vi "NavbalLabVIEW(15-5-21).vi"() -> ()   [LabVIEW 2010] (continued)
              n357 = Array Size(array=w4216) -> (size(s)=w4217:i32[])
              n358 = Array Size(array=w4219) -> (size(s)=w4222:i32[])
              n359 = Index Array(array=w4217, index=1) -> (element=w4215:i32)
              n360 = Index Array(array=w4222, index=1) -> (element=w4220:i32)
              n361 = Insert Into Array(array=w4219, index (dim 1)=w4220, new element=w4223) -> (w4210:dbl[][][])  [unwired: 2 in]
              n362 = Insert Into Array(array=w4216, index (dim 1)=w4215, new element=w4214) -> (w4209:dbl[][][])  [unwired: 2 in]
              n363 = Array Size(array=w4210) -> (size(s)=w4213:i32[])
              n364 = Index Array(array=w4213, index=1) -> (element=w4211:i32)
              n365 = Insert Into Array(array=w4210, index (dim 1)=w4211, new element=w4209) -> (w4208:dbl[][][])  [unwired: 2 in]
            }
          }
          n366 = Array Size(array=w3330) -> (size(s)=w3436:i32[])
          n367 = Array Size(array=w3333) -> (size(s)=w3427:i32[])
          n368 = Array Size(array=w3332) -> (size(s)=w3425:i32[])
          n369 = Array Size(array=w3331) -> (size(s)=w3420:i32[])
          n370 = Index Array(array=w3436, index=0) -> (element=w3418:i32)
          n371 = Index Array(array=w3427, index=0) -> (element=w3426:i32)
          n372 = Index Array(array=w3425, index=0) -> (element=w3423:i32)
          n373 = Index Array(array=w3420, index=0) -> (element=w3419:i32)
          n374 = Greater?(x=w3418, y=700) -> (0:w3429:bool)
          n375 = Or(x="Mark Current", y=w3366) -> (x .or. y?=w3367:bool)
          n376 = case shown="True" "Averaging" {
            tunnel: [10 "Number of Averages"] -> w3416
            frame False {
            }
            frame True {
            }
          }
          n377 = case shown="\"Simulated Signals Ohio\"" w3369 {
            tunnel: [w4378 w4427 w4476] -> w3480
            tunnel: [w4382 w4431 w4480] -> w3478
            tunnel: [w4380 w4429 w4478] -> w3523
            tunnel: [w4369 w4424 w4473] -> w3328
            tunnel: [w4381 w4430 w4479] -> w3407
            tunnel: [w4379 w4428 w4477] -> w3406
            tunnel: [w4377 w4426 w4475] -> w3456
            tunnel: [w4376 w4425 w4474] -> w3532
            tunnel: w3530 -> [w4383 w4432 w4481]
            tunnel: w3416 -> [w4370 w4418 w4467]
            frame "Simulated Signals Ohio" {
              # "Ensure that buffer is full before processing"
              # ">>  data out from buffer  >>"
              n378 = local read "Number of Samples"() -> (w4384:i32)
              n379 = call "Convert to Dynamic Data11"("Array"=bool[] [FALSE, FALSE, FALSE, FALSE, FALSE, FALSE, FALSE, FALSE, FALSE, FALSE, TRUE, FALSE, FALSE, FALSE, FALSE, FALSE, FALSE, FALSE, FALSE, FALSE]) -> ("Dynamic Data Type"=w4372:dynamicdata)  [unwired: 3 in]
              n380 = call-poly <userlib>:"Circular Buffer.vi"("Buffer Size"=w4383, "Read Size"=w4384, "Operation"=Circular_Buffer_Operations."Read (most recent)") -> ("Data Out"=w4371:waveform(dbl)[])  [unwired: 5 in, 3 out]
              n381 = call "Select Tach Port2"("Selector Input"=w4372, "Signals"=w4371) -> ("Signal Out"=w4376:dynamicdata)  [unwired: 8 in, 1 out]
              n382 = call "Convert from Dynamic Data49"("Dynamic Data Type"=w4371) -> ("Array"=w4387:dbl[][])  [unwired: 3 in]
              n383 = call "Convert to Dynamic Data10"("Array"=bool[] [TRUE, FALSE, FALSE, FALSE, FALSE, FALSE, FALSE, FALSE, FALSE, FALSE, FALSE, FALSE, FALSE, FALSE, FALSE, FALSE, FALSE, FALSE, FALSE, FALSE]) -> ("Dynamic Data Type"=w4374:dynamicdata)  [unwired: 3 in]
              n384 = Array Size(array=w4387) -> (size(s)=w4390:i32[])
              n385 = call "Select Tach Stbd3"("Selector Input"=w4374, "Signals"=w4371) -> ("Signal Out"=w4369:dynamicdata)  [unwired: 8 in, 1 out]
              n386 = Equal?(x=w4390, y=w4384) -> (x = y?=w4388:bool[])
              n387 = Index Array(array=w4388, index=1) -> (element=w4385:bool)
              n388 = case shown="True" w4385 {
                tunnel: w4371 -> [_ w4410]
                tunnel: [w4391 w4403] -> w4382
                tunnel: [w4393 w4400] -> w4381
                tunnel: [w4391 w4402] -> w4380
                tunnel: [w4391 w4401] -> w4378
                tunnel: [w4393 w4397] -> w4379
                tunnel: [w4393 w4398] -> w4377
                tunnel: w4370 -> [_ w4396]
                frame False {
                  w4391 = cluster{"x0":dbl, "dx":dbl, "magnitude":dbl[]}[] [] ("spectra")
                  n389 = local read "DAQ Start"() -> (w4392:bool)
                  n390 = case shown="True" w4392 {
                    frame False {
                      n391 = property on="DAQ Start" class="Bool (strict)"("BoolText.Text"="DAQ START" ("Boolean Text.Text")) -> ()  [unwired: 2 in, 2 out]
                    }
                    frame True {
                      n392 = property on="DAQ Start" class="Bool (strict)"("BoolText.Text"="Buffering..." ("Boolean Text.Text")) -> ()  [unwired: 2 in, 2 out]
                    }
                  }
                  n393 = local read "Default Stbd Graph"() -> (w4393:dynamicdata)
                }
                frame True {
                  # "convert to VdB"
                  # "convert to VdB"
                  # "convert to VdB"
                  n394 = local read "DAQ Start"() -> (w4399:bool)
                  n395 = case shown="True" w4399 {
                    frame False {
                    }
                    frame True {
                      n396 = property on="DAQ Start" class="Bool (strict)"("BoolText.Text"="DAQ STOP" ("Boolean Text.Text")) -> ()  [unwired: 2 in, 2 out]
                    }
                  }
                  n397 = call "Convert to Dynamic Data3"("Array"=bool[] [FALSE, FALSE, FALSE, FALSE, FALSE, FALSE, FALSE, FALSE, FALSE, FALSE, TRUE, TRUE, TRUE, TRUE, TRUE, TRUE, TRUE, TRUE, TRUE, TRUE]) -> ("Dynamic Data Type"=w4411:dynamicdata)  [unwired: 3 in]
                  n398 = call "Select Port"("Selector Input"=w4411, "Signals"=w4410) -> ("Signal Out"=w4397:dynamicdata)  [unwired: 8 in, 1 out]
                  n399 = call "Convert to Dynamic Data2"("Array"=bool[] [TRUE, TRUE, TRUE, TRUE, TRUE, TRUE, TRUE, TRUE, TRUE, TRUE, FALSE, FALSE, FALSE, FALSE, FALSE, FALSE, FALSE, FALSE, FALSE, FALSE]) -> ("Dynamic Data Type"=w4415:dynamicdata)  [unwired: 3 in]
                  n400 = call "Select Stbd"("Selector Input"=w4415, "Signals"=w4410) -> ("Signal Out"=w4400:dynamicdata)  [unwired: 8 in, 1 out]
                  n401 = call "Convert to Dynamic Data4"("Array"=bool[] [FALSE, FALSE, FALSE, FALSE, FALSE, FALSE, FALSE, FALSE, FALSE, FALSE, FALSE, FALSE, FALSE, FALSE, FALSE, FALSE, FALSE, FALSE, FALSE, FALSE, TRUE, TRUE, TRUE, TRUE, TRUE, TRUE, TRUE, TRUE, TRUE, TRUE, TRUE, TRUE]) -> ("Dynamic Data Type"=w4412:dynamicdata)  [unwired: 3 in]
                  n402 = call "Select Corner"("Selector Input"=w4412, "Signals"=w4410) -> ("Signal Out"=w4398:dynamicdata)  [unwired: 8 in, 1 out]
                  n403 = call-poly <vilib>:"SVL Set dB Reference.vi"("dB reference [EU]"=3.937e-07, "scaled signals in [EU]"=w4400) -> ("scaled signals out [EU]"=w4408:waveform(dbl)[])  [unwired: 8 in, 1 out]
                  n404 = call-poly <vilib>:"SVL Set dB Reference.vi"("dB reference [EU]"=3.937e-07, "scaled signals in [EU]"=w4398) -> ("scaled signals out [EU]"=w4404:waveform(dbl)[])  [unwired: 8 in, 1 out]
                  n405 = call-poly <vilib>:"SVL Set dB Reference.vi"("dB reference [EU]"=3.937e-07, "scaled signals in [EU]"=w4397) -> ("scaled signals out [EU]"=w4406:waveform(dbl)[])  [unwired: 8 in, 1 out]
                  n406 = call "Power Spectrum3"("input signals"=w4406, "number of averages"=w4396) -> ("spectra"=w4402:cluster{"x0":dbl, "dx":dbl, "magnitude":dbl[]}[])  [unwired: 12 in, 5 out]
                  n407 = call "Power Spectrum6"("input signals"=w4404, "number of averages"=w4396) -> ("spectra"=w4401:cluster{"x0":dbl, "dx":dbl, "magnitude":dbl[]}[])  [unwired: 12 in, 5 out]
                  n408 = call "Power Spectrum2"("input signals"=w4408, "number of averages"=w4396) -> ("spectra"=w4403:cluster{"x0":dbl, "dx":dbl, "magnitude":dbl[]}[])  [unwired: 12 in, 5 out]
                }
              }
            }
            frame "LA Class" {
              # "Ensure that buffer is full before processing"
              # ">>  data out from buffer  >>"
              n409 = local read "Number of Samples"() -> (w4433:i32)
              n410 = call "Convert to Dynamic Data19"("Array"=bool[] [FALSE, FALSE, FALSE, FALSE, FALSE, FALSE, FALSE, FALSE, FALSE, FALSE, FALSE, FALSE, FALSE, FALSE, FALSE, FALSE, FALSE, FALSE, FALSE, FALSE, FALSE, FALSE, FALSE, FALSE, FALSE, TRUE]) -> ("Dynamic Data Type"=w4420:dynamicdata)  [unwired: 3 in]
              n411 = call-poly <userlib>:"Circular Buffer.vi"("Buffer Size"=w4432, "Read Size"=w4433, "Operation"=Circular_Buffer_Operations."Read (most recent)") -> ("Data Out"=w4419:waveform(dbl)[])  [unwired: 5 in, 3 out]
              n412 = call "Select Tach Port4"("Selector Input"=w4420, "Signals"=w4419) -> ("Signal Out"=w4425:dynamicdata)  [unwired: 8 in, 1 out]
              n413 = call "Convert from Dynamic Data5"("Dynamic Data Type"=w4419) -> ("Array"=w4436:dbl[][])  [unwired: 3 in]
              n414 = call "Convert to Dynamic Data18"("Array"=bool[] [TRUE, FALSE, FALSE, FALSE, FALSE, FALSE, FALSE, FALSE, FALSE, FALSE, FALSE, FALSE, FALSE, FALSE, FALSE, FALSE, FALSE, FALSE, FALSE, FALSE]) -> ("Dynamic Data Type"=w4422:dynamicdata)  [unwired: 3 in]
              n415 = Array Size(array=w4436) -> (size(s)=w4439:i32[])
              n416 = call "Select Tach Stbd2"("Selector Input"=w4422, "Signals"=w4419) -> ("Signal Out"=w4424:dynamicdata)  [unwired: 8 in, 1 out]
              n417 = Equal?(x=w4439, y=w4433) -> (x = y?=w4437:bool[])
              n418 = Index Array(array=w4437, index=1) -> (element=w4434:bool)
              n419 = case shown="False" w4434 {
                tunnel: w4419 -> [_ w4462]
                tunnel: [w4440 w4455] -> w4431
                tunnel: [w4442 w4452] -> w4430
                tunnel: [w4440 w4454] -> w4429
                tunnel: [w4440 w4453] -> w4427
                tunnel: [w4442 w4449] -> w4428
                tunnel: [w4442 w4450] -> w4426
                tunnel: w4418 -> [_ w4448]
                frame False {
                  w4440 = cluster{"x0":dbl, "dx":dbl, "magnitude":dbl[]}[] [] ("spectra")
                  n420 = local read "DAQ Start"() -> (w4441:bool)
                  n421 = case shown="True" w4441 {
                    frame False {
                      n422 = property on="DAQ Start" class="Bool (strict)"("BoolText.Text"="DAQ START" ("Boolean Text.Text")) -> ()  [unwired: 2 in, 2 out]
                    }
                    frame True {
                      n423 = property on="DAQ Start" class="Bool (strict)"("BoolText.Text"="Buffering..." ("Boolean Text.Text")) -> ()  [unwired: 2 in, 2 out]
                    }
                  }
                  n424 = local read "Default Stbd Graph"() -> (w4442:dynamicdata)
                }
                frame True {
                  # "convert to VdB"
                  # "convert to VdB"
                  # "convert to VdB"
                  n425 = local read "DAQ Start"() -> (w4451:bool)
                  n426 = case shown="True" w4451 {
                    frame False {
                    }
                    frame True {
                      n427 = property on="DAQ Start" class="Bool (strict)"("BoolText.Text"="DAQ STOP" ("Boolean Text.Text")) -> ()  [unwired: 2 in, 2 out]
                    }
                  }
                  n428 = call "Convert to Dynamic Data16"("Array"=bool[] [FALSE, FALSE, FALSE, FALSE, FALSE, FALSE, FALSE, FALSE, FALSE, FALSE, FALSE, FALSE, FALSE, FALSE, FALSE, FALSE, FALSE, FALSE, FALSE, FALSE, FALSE, FALSE, FALSE, FALSE, FALSE, TRUE, TRUE, TRUE, TRUE, TRUE, TRUE, TRUE, TRUE, TRUE, TRUE, TRUE, TRUE, TRUE]) -> ("Dynamic Data Type"=w4463:dynamicdata)  [unwired: 3 in]
                  n429 = call "Select Port3"("Selector Input"=w4463, "Signals"=w4462) -> ("Signal Out"=w4449:dynamicdata)  [unwired: 8 in, 1 out]
                  n430 = call "Convert to Dynamic Data15"("Array"=bool[] [TRUE, FALSE, FALSE, FALSE, FALSE, FALSE, FALSE, FALSE, FALSE, FALSE, FALSE, FALSE, FALSE, TRUE, TRUE, TRUE, TRUE, TRUE, TRUE, TRUE, TRUE, TRUE, TRUE, TRUE, TRUE, FALSE, FALSE, FALSE, FALSE, FALSE, FALSE, FALSE, FALSE, FALSE, FALSE, FALSE, FALSE, FALSE]) -> ("Dynamic Data Type"=w4465:dynamicdata)  [unwired: 3 in]
                  n431 = call "Select Stbd4"("Selector Input"=w4465, "Signals"=w4462) -> ("Signal Out"=w4452:dynamicdata)  [unwired: 8 in, 1 out]
                  n432 = call "Convert to Dynamic Data17"("Array"=bool[] [FALSE, TRUE, TRUE, TRUE, TRUE, TRUE, TRUE, TRUE, TRUE, TRUE, TRUE, TRUE, TRUE, FALSE, FALSE, FALSE, FALSE, FALSE, FALSE, FALSE, FALSE, FALSE, FALSE, FALSE, FALSE, FALSE, FALSE, FALSE, FALSE, FALSE, FALSE, FALSE, FALSE, FALSE, FALSE, FALSE, FALSE, FALSE]) -> ("Dynamic Data Type"=w4464:dynamicdata)  [unwired: 3 in]
                  n433 = call "Select Corner4"("Selector Input"=w4464, "Signals"=w4462) -> ("Signal Out"=w4450:dynamicdata)  [unwired: 8 in, 1 out]
                  n434 = call-poly <vilib>:"SVL Set dB Reference.vi"("dB reference [EU]"=3.937e-07, "scaled signals in [EU]"=w4452) -> ("scaled signals out [EU]"=w4460:waveform(dbl)[])  [unwired: 8 in, 1 out]
                  n435 = call-poly <vilib>:"SVL Set dB Reference.vi"("dB reference [EU]"=3.937e-07, "scaled signals in [EU]"=w4450) -> ("scaled signals out [EU]"=w4456:waveform(dbl)[])  [unwired: 8 in, 1 out]
                  n436 = call-poly <vilib>:"SVL Set dB Reference.vi"("dB reference [EU]"=3.937e-07, "scaled signals in [EU]"=w4449) -> ("scaled signals out [EU]"=w4458:waveform(dbl)[])  [unwired: 8 in, 1 out]
                  n437 = call "Power Spectrum12"("input signals"=w4456, "number of averages"=w4448) -> ("spectra"=w4453:cluster{"x0":dbl, "dx":dbl, "magnitude":dbl[]}[])  [unwired: 12 in, 5 out]
                  n438 = call "Power Spectrum11"("input signals"=w4458, "number of averages"=w4448) -> ("spectra"=w4454:cluster{"x0":dbl, "dx":dbl, "magnitude":dbl[]}[])  [unwired: 12 in, 5 out]
                  n439 = call "Power Spectrum10"("input signals"=w4460, "number of averages"=w4448) -> ("spectra"=w4455:cluster{"x0":dbl, "dx":dbl, "magnitude":dbl[]}[])  [unwired: 12 in, 5 out]
                }
              }
            }
            frame "Ohio Class" {
              # "Ensure that buffer is full before processing"
              # ">>  data out from buffer  >>"
              n440 = local read "Number of Samples"() -> (w4482:i32)
              n441 = call "Convert to Dynamic Data24"("Array"=bool[] [FALSE, FALSE, FALSE, FALSE, FALSE, FALSE, FALSE, FALSE, FALSE, FALSE, FALSE, FALSE, FALSE, FALSE, FALSE, FALSE, FALSE, FALSE, FALSE, FALSE, FALSE, FALSE, TRUE]) -> ("Dynamic Data Type"=w4469:dynamicdata)  [unwired: 3 in]
              n442 = call-poly <userlib>:"Circular Buffer.vi"("Buffer Size"=w4481, "Read Size"=w4482, "Operation"=Circular_Buffer_Operations."Read (most recent)") -> ("Data Out"=w4468:waveform(dbl)[])  [unwired: 5 in, 3 out]
              n443 = call "Select Tach Port5"("Selector Input"=w4469, "Signals"=w4468) -> ("Signal Out"=w4474:dynamicdata)  [unwired: 8 in, 1 out]
              n444 = call "Convert from Dynamic Data6"("Dynamic Data Type"=w4468) -> ("Array"=w4485:dbl[][])  [unwired: 3 in]
              n445 = call "Convert to Dynamic Data23"("Array"=bool[] [TRUE, FALSE, FALSE, FALSE, FALSE, FALSE, FALSE, FALSE, FALSE, FALSE, FALSE, FALSE, FALSE, FALSE, FALSE, FALSE, FALSE, FALSE, FALSE, FALSE]) -> ("Dynamic Data Type"=w4471:dynamicdata)  [unwired: 3 in]
              n446 = Array Size(array=w4485) -> (size(s)=w4488:i32[])
              n447 = call "Select Tach Stbd5"("Selector Input"=w4471, "Signals"=w4468) -> ("Signal Out"=w4473:dynamicdata)  [unwired: 8 in, 1 out]
              n448 = Equal?(x=w4488, y=w4482) -> (x = y?=w4486:bool[])
              n449 = Index Array(array=w4486, index=1) -> (element=w4483:bool)
              n450 = case shown="False" w4483 {
                tunnel: w4468 -> [_ w4508]
                tunnel: [w4489 w4501] -> w4480
                tunnel: [w4491 w4498] -> w4479
                tunnel: [w4489 w4500] -> w4478
                tunnel: [w4489 w4499] -> w4476
                tunnel: [w4491 w4495] -> w4477
                tunnel: [w4491 w4496] -> w4475
                tunnel: w4467 -> [_ w4494]
                frame False {
                  w4489 = cluster{"x0":dbl, "dx":dbl, "magnitude":dbl[]}[] [] ("spectra")
                  n451 = local read "DAQ Start"() -> (w4490:bool)
                  n452 = case shown="True" w4490 {
                    frame False {
                      n453 = property on="DAQ Start" class="Bool (strict)"("BoolText.Text"="DAQ START" ("Boolean Text.Text")) -> ()  [unwired: 2 in, 2 out]
                    }
                    frame True {
                      n454 = property on="DAQ Start" class="Bool (strict)"("BoolText.Text"="Buffering..." ("Boolean Text.Text")) -> ()  [unwired: 2 in, 2 out]
                    }
                  }
                  n455 = local read "Default Stbd Graph"() -> (w4491:dynamicdata)
                }
                frame True {
                  # "convert to VdB"
                  # "convert to VdB"
                  # "convert to VdB"
                  n456 = local read "DAQ Start"() -> (w4497:bool)
                  n457 = case shown="True" w4497 {
                    frame False {
                    }
                    frame True {
                      n458 = property on="DAQ Start" class="Bool (strict)"("BoolText.Text"="DAQ STOP" ("Boolean Text.Text")) -> ()  [unwired: 2 in, 2 out]
                    }
                  }
                  n459 = call "Convert to Dynamic Data21"("Array"=bool[] [FALSE, FALSE, FALSE, FALSE, FALSE, FALSE, FALSE, FALSE, FALSE, FALSE, FALSE, FALSE, FALSE, FALSE, FALSE, FALSE, FALSE, FALSE, FALSE, FALSE, FALSE, FALSE, TRUE, TRUE, TRUE, TRUE, TRUE, TRUE, TRUE, TRUE, TRUE, TRUE]) -> ("Dynamic Data Type"=w4509:dynamicdata)  [unwired: 3 in]
                  n460 = call "Select Port5"("Selector Input"=w4509, "Signals"=w4508) -> ("Signal Out"=w4495:dynamicdata)  [unwired: 8 in, 1 out]
                  n461 = call "Convert to Dynamic Data20"("Array"=bool[] [TRUE, FALSE, FALSE, FALSE, FALSE, FALSE, FALSE, FALSE, FALSE, FALSE, FALSE, FALSE, FALSE, TRUE, TRUE, TRUE, TRUE, TRUE, TRUE, TRUE, TRUE, TRUE]) -> ("Dynamic Data Type"=w4513:dynamicdata)  [unwired: 3 in]
                  n462 = call "Select Stbd5"("Selector Input"=w4513, "Signals"=w4508) -> ("Signal Out"=w4498:dynamicdata)  [unwired: 8 in, 1 out]
                  n463 = call "Convert to Dynamic Data22"("Array"=bool[] [FALSE, TRUE, TRUE, TRUE, TRUE, TRUE, TRUE, TRUE, TRUE, TRUE, TRUE, TRUE, TRUE, FALSE, FALSE, FALSE, FALSE, FALSE, FALSE, FALSE, FALSE, FALSE, FALSE, FALSE, FALSE, FALSE, FALSE, FALSE, FALSE, FALSE, FALSE, FALSE]) -> ("Dynamic Data Type"=w4510:dynamicdata)  [unwired: 3 in]
                  n464 = call "Select Corner5"("Selector Input"=w4510, "Signals"=w4508) -> ("Signal Out"=w4496:dynamicdata)  [unwired: 8 in, 1 out]
                  n465 = call-poly <vilib>:"SVL Set dB Reference.vi"("dB reference [EU]"=3.937e-07, "scaled signals in [EU]"=w4498) -> ("scaled signals out [EU]"=w4506:waveform(dbl)[])  [unwired: 8 in, 1 out]
                  n466 = call-poly <vilib>:"SVL Set dB Reference.vi"("dB reference [EU]"=3.937e-07, "scaled signals in [EU]"=w4496) -> ("scaled signals out [EU]"=w4502:waveform(dbl)[])  [unwired: 8 in, 1 out]
                  n467 = call-poly <vilib>:"SVL Set dB Reference.vi"("dB reference [EU]"=3.937e-07, "scaled signals in [EU]"=w4495) -> ("scaled signals out [EU]"=w4504:waveform(dbl)[])  [unwired: 8 in, 1 out]
                  n468 = call "Power Spectrum15"("input signals"=w4502, "number of averages"=w4494) -> ("spectra"=w4499:cluster{"x0":dbl, "dx":dbl, "magnitude":dbl[]}[])  [unwired: 12 in, 5 out]
                  n469 = call "Power Spectrum13"("input signals"=w4506, "number of averages"=w4494) -> ("spectra"=w4501:cluster{"x0":dbl, "dx":dbl, "magnitude":dbl[]}[])  [unwired: 12 in, 5 out]
                  n470 = call "Power Spectrum14"("input signals"=w4504, "number of averages"=w4494) -> ("spectra"=w4500:cluster{"x0":dbl, "dx":dbl, "magnitude":dbl[]}[])  [unwired: 12 in, 5 out]
                }
              }
            }
          }
          "Default Stbd Graph" <- w3407
          "spectra" <- w3523
          n471 = call "Convert from Dynamic Data48"("Dynamic Data Type"=w3532) -> ("Array"=w3544:dbl[])  [unwired: 3 in]
          n472 = Array Max & Min(array=w3544) -> (max value=w3533:dbl)  [unwired: 3 out]
          n473 = Greater?(x=w3533, y=1.0) -> (0:w3542:bool)
          n474 = case shown="True" w3542 {
            tunnel: w3532 -> [_ w4359]
            tunnel: [0.0 ("detected frequency") w4356] -> w3538
            frame False {
            }
            frame True {
              n475 = call "Filter2"("Signal"=w4359) -> ("Filtered Signal"=w4360:dynamicdata)  [unwired: 9 in, 1 out]
              n476 = call-poly <vilib>:"Extract Single Tone Information.vi"("time signals in"=w4360) -> ("detected frequencies"=w4358:dbl[])  [unwired: 5 in, 5 out]
              n477 = Index Array(array=w4358, index=0) -> (element=w4356:dbl)
            }
          }
          "Frequency (Hz) 2" <- w3538
          n478 = Multiply(x=w3538, y=60.0) -> (x*y=→"Frequency (RPM) 2":dbl)
          n479 = In Range and Coerce(upper limit=60.6, x=w3538, lower limit=60.4) -> (In Range?=w3535:bool)  [unwired: 1 out]
          n480 = case shown="True" w3535 {
            tunnel: [u32 16752008 u32 5308226] -> w3534
            frame False {
            }
            frame True {
            }
          }
          n481 = property on="Frequency (Hz) 2" class="DigNum (strict)"("NumText.BGColor"=w3534) -> ()  [unwired: 2 in, 2 out]
          n482 = property on="Frequency (RPM) 2" class="DigNum (strict)"("NumText.BGColor"=w3534) -> ()  [unwired: 2 in, 2 out]
          n483 = call "Convert from Dynamic Data47"("Dynamic Data Type"=w3328) -> ("Array"=w3554:dbl[])  [unwired: 3 in]
          n484 = Array Max & Min(array=w3554) -> (max value=w3551:dbl)  [unwired: 3 out]
          n485 = Greater?(x=w3551, y=1.0) -> (0:w3552:bool)
          n486 = case shown="True" w3552 {
            tunnel: w3328 -> [_ w4365]
            tunnel: [0.0 ("detected frequency") w4364] -> w3537
            frame False {
            }
            frame True {
              n487 = call "Filter"("Signal"=w4365) -> ("Filtered Signal"=w4366:dynamicdata)  [unwired: 9 in, 1 out]
              n488 = call-poly <vilib>:"Extract Single Tone Information.vi"("time signals in"=w4366) -> ("detected frequencies"=w4367:dbl[])  [unwired: 5 in, 5 out]
              n489 = Index Array(array=w4367, index=0) -> (element=w4364:dbl)
            }
          }
          "Frequency (Hz) 1" <- w3537
          n490 = Multiply(x=w3537, y=60.0) -> (x*y=→"Frequency (RPM) 1":dbl)
          n491 = In Range and Coerce(upper limit=59.6, x=w3537, lower limit=59.4) -> (In Range?=w3549:bool)  [unwired: 1 out]
          n492 = case shown="True" w3549 {
            tunnel: [u32 16752008 u32 5308226] -> w3545
            frame False {
            }
            frame True {
            }
          }
          n493 = property on="Frequency (Hz) 1" class="DigNum (strict)"("NumText.BGColor"=w3545) -> ()  [unwired: 2 in, 2 out]
          n494 = property on="Frequency (RPM) 1" class="DigNum (strict)"("NumText.BGColor"=w3545) -> ()  [unwired: 2 in, 2 out]
          n495 = case shown="True" w3367 {
            frame False {
            }
            frame True {
              n496 = local read "time string"() -> (→"Marker Time":string)
              n497 = local read "Mils/Sec-Phase(CORNERS-Stbd)"() -> (w4242:sgl[][])
              n498 = local read "Mils/Sec-Phase(CORNERS-Port)"() -> (w4245:sgl[][])
              n499 = local read "Mils/Sec-Phase(STBD)"() -> (w4244:dbl[][])
              n500 = local read "Mils/Sec-Phase(PORT)"() -> (w4243:sgl[][])
              n501 = Array Size(array=w4242) -> (size(s)=w4241:i32[])
              n502 = Index Array(array=w4241, index=0) -> (element=w4239:i32)
              n503 = Insert Into Array(array=w4242, index (row)=w4239, new element #1=w4245, new element #2=w4244, new element #3=w4243) -> (w4238:sgl[][])  [unwired: 1 in]
              n504 = local read "Marker Mag"() -> (w4234:sgl[][])
              n505 = local read "Marker Phase"() -> (w4227:sgl[][])
              n506 = Index Array "Mag"(array=w4238, index (col)=0 ("disabled index (col)")) -> (element=w4235:sgl[])  [unwired: 1 in]
              n507 = Index Array "Phase"(array=w4238, index (col)=1 ("disabled index (col)")) -> (element=w4226:sgl[])  [unwired: 1 in]
              n508 = Array Size(array=w4234) -> (size(s)=w4233:i32[])
              n509 = Array Size(array=w4227) -> (size(s)=w4228:i32[])
              n510 = Index Array(array=w4233, index=1) -> (element=w4231:i32)
              n511 = Insert Into Array(array=w4234, index (col)=w4231, new element=w4235) -> (→"Marker Mag":sgl[][])  [unwired: 1 in]
              n512 = Index Array(array=w4228, index=1) -> (element=w4225:i32)
              n513 = Insert Into Array(array=w4227, index (col)=w4225, new element=w4226) -> (→"Marker Phase":sgl[][])  [unwired: 1 in]
            }
          }
          n514 = case shown="True" w3429 {
            tunnel: [w3940 w3944] -> w3434
            tunnel: w3333 -> [w3940 w3957]
            tunnel: [w3939 w3943] -> w3433
            tunnel: w3332 -> [w3939 w3955]
            tunnel: [w3938 w3942] -> w3432
            tunnel: w3331 -> [w3938 w3950]
            tunnel: [w3937 w3941] -> w3431
            tunnel: w3330 -> [w3937 w3948]
            tunnel: w3426 -> [_ w3956]
            tunnel: w3423 -> [_ w3954]
            tunnel: 600 ("y") -> [_ w3945]
            tunnel: w3419 -> [_ w3951]
            tunnel: w3418 -> [_ w3947]
            frame False {
            }
            frame True {
              n515 = Subtract(x=w3956, y=w3945) -> (x-y=w3953:i32)
              n516 = Subtract(x=w3954, y=w3945) -> (x-y=w3952:i32)
              n517 = Subtract(x=w3951, y=w3945) -> (x-y=w3949:i32)
              n518 = Subtract(x=w3947, y=w3945) -> (x-y=w3946:i32)
              n519 = Delete From Array(array=w3957, length=w3953, index (dim 0)=w3945) -> (array with subset deleted=w3944:dbl[][][])  [unwired: 2 in, 1 out]
              n520 = Delete From Array(array=w3955, length=w3952, index (dim 0)=w3945) -> (array with subset deleted=w3943:dbl[][][])  [unwired: 2 in, 1 out]
              n521 = Delete From Array(array=w3950, length=w3949, index (dim 0)=w3945) -> (array with subset deleted=w3942:dbl[][][])  [unwired: 2 in, 1 out]
              n522 = Delete From Array(array=w3948, length=w3946, index (dim 0)=w3945) -> (array with subset deleted=w3941:dbl[][][])  [unwired: 2 in, 1 out]
            }
          }
          n523 = Array Subset(array=w3334, index (dim 0)=0 ("index"), length (dim 0)=600 ("length"), index (dim 1)="DAQ Listbox", length (dim 1)=1 ("length"), index (dim 2)=0 ("index"), length (dim 2)=2 ("length")) -> (w3610:dbl[][][])
          n524 = Array Subset(array=w3334, index (dim 0)=0 ("index"), length (dim 0)=1 ("length"), index (dim 1)="DAQ Listbox", length (dim 1)=1 ("length"), index (dim 2)=0 ("index"), length (dim 2)=2 ("length")) -> (w3595:dbl[][][])
          n525 = Reshape Array(w3610, 600 ("dimension size"), 2 ("dimension size")) -> (w3572:dbl[][])
          n526 = Reshape Array(w3595, 1 ("dimension size"), 2 ("dimension size")) -> (w3582:dbl[][])
          n527 = Index Array(array=w3582, index (col)=0 ("disabled index (col)")) -> (element=w3584:dbl[])  [unwired: 1 in]
          n528 = Index Array(array=w3582, index (col)=1 ("disabled index (col)")) -> (element=w3581:dbl[])  [unwired: 1 in]
          n529 = Array Subset(array=w3572, index (row)=0 ("index"), length (row)=600 ("length"), index (col)=0 ("index"), length (col)=1 ("length")) -> (w3573:dbl[][])
          n530 = Array Subset(array=w3572, index (row)=0 ("index"), length (row)=600 ("length"), index (col)=1 ("index"), length (col)=1 ("length")) -> (w3597:dbl[][])
          n531 = Reshape Array(w3584, 1 ("dimension size")) -> (w3585:dbl[])
          n532 = Reshape Array(w3581, 1 ("dimension size")) -> (w3591:dbl[])
          n533 = Index Array(array=w3585, index=0) -> (element=w3579:dbl)
          n534 = Index Array(array=w3591, index=0) -> (element=w3616:dbl)
          n535 = Reshape Array(w3597, 600 ("dimension size")) -> (w3576:dbl[])
          n536 = Reshape Array(w3573, 600 ("dimension size")) -> (w3580:dbl[])
          n537 = Insert Into Array(array=w3580, index=0, new element=w3579) -> (→"mag":dbl[])
          n538 = Insert Into Array(array=w3576, index=0, new element=w3616) -> (→"phase":dbl[])
          n539 = property on="Tab 3" class="TabCtl (strict)"() -> ("Visible"=w3443:bool)  [unwired: 2 in, 2 out]
          n540 = property on="Tab 3" class="TabCtl (strict)"() -> ("Value"=w3446:T9)  [unwired: 2 in, 2 out]
          n541 = Equal?(x=w3446, y=T19."Step 6: Polar Plots") -> (x = y?=w3444:bool)
          n542 = And(x=w3444, y=w3443) -> (x .and. y?=w3442:bool)
          n543 = case shown="True" w3442 {
            frame False {
            }
            frame True {
              w3989 = 0 ("index")
              w4002 = T21."Application Font" ("desired font(Application)")
              w4004 = cluster{"width":i16, "height":i16} {"width"=575, "height"=575} ("dimensions (w,h)")
              # "Find the max magnitude to be plotted,\nand adjust the scaling of all plots"
              # "Add Corresponding Prediction measurement to Polar plot"
              # "Add Corresponding Baseline measurement to Polar plot"
              # "Polar Plot"
              n544 = local read "Marker Phase"() -> (w3970:sgl[][])
              n545 = local read "Pred plot"() -> (w3958:dbl[][])
              n546 = local read "Marker Mag"() -> (w3963:sgl[][])
              n547 = Array Size(array=w3963) -> (size(s)=w3966:i32[])
              n548 = local read "Ref Pt Plot"() -> (w3976:sgl[][])
              n549 = Index Array(array=w3966, index=1) -> (element=w3964:i32)
              n550 = local read "DAQ Listbox"() -> (w3969:i32)
              n551 = Index Array(array=w3958, index (col)=1 ("disabled index (col)")) -> (element=w3959:dbl[])  [unwired: 1 in]
              n552 = Index Array(array=w3958, index (col)=0 ("disabled index (col)")) -> (element=w3960:dbl[])  [unwired: 1 in]
              n553 = for {
                N: w3964 -> [_]
                tunnel: [w4013] -> w3968
                tunnel: [w4015] -> w3967 mode=indexing
                tunnel: w3969 -> [w4014]
                tunnel: w3970 -> [w4008]
                tunnel: w3963 -> [w4007]
                i -> [w4011]
                n554 = Index Array(array=w4007, index (row)=w4014) -> (element=w4013:sgl[])  [unwired: 1 in]
                n555 = Index Array(array=w4008, index (row)=w4014) -> (element=w4012:sgl[])  [unwired: 1 in]
                n556 = Index Array(array=w4012, index=w4011) -> (element=w4009:sgl)
                n557 = Index Array(array=w4013, index=w4011) -> (element=w4010:sgl)
                n558 = Bundle(w4010, w4009) -> (w4015:cluster{sgl, sgl})  [unwired: 1 in]
              }
              n559 = Index Array(array=w3976, index (col)=0 ("disabled index (col)")) -> (element=w3978:sgl[])  [unwired: 1 in]
              n560 = Index Array(array=w3976, index (col)=1 ("disabled index (col)")) -> (element=w3975:sgl[])  [unwired: 1 in]
              n561 = Index Array(array=w3959, index=w3969) -> (element=w3991:dbl)
              n562 = Index Array(array=w3960, index=w3969) -> (element=w3988:dbl)
              n563 = for {
                N: 600 -> [_]
                tunnel: [w4020] -> w4003 mode=indexing
                i -> [w4021]
                n564 = local read "phase"() -> (w4016:dbl[])
                n565 = local read "mag"() -> (w4017:dbl[])
                n566 = Index Array(array=w4017, index=w4021) -> (element=w4019:dbl)
                n567 = Index Array(array=w4016, index=w4021) -> (element=w4018:dbl)
                n568 = Bundle("mag. (Vpeak)"=w4019, "mag. (Vpeak)"=w4018) -> (w4020:cluster{"mag. (Vpeak)":dbl, "mag. (Vpeak)":dbl})  [unwired: 1 in]
              }
              n569 = local read "mag"() -> (w3994:dbl[])
              n570 = Bundle("Real Matrix Element"=w3988, "Real Matrix Element"=w3991) -> (w3983:T22)  [unwired: 1 in]
              n571 = Index Array(array=w3978, index=w3969) -> (element=w3993:sgl)
              n572 = Index Array(array=w3975, index=w3969) -> (element=w3997:sgl)
              n573 = Insert Into Array(array=w3994, index=w3989, new element #1=w3993, new element #2=0 ("new element/subarray"), new element #3=w3968) -> (w3990:dbl[])
              n574 = Bundle(w3993, w3997) -> (w3996:cluster{sgl, sgl})  [unwired: 1 in]
              n575 = Initialize Array(w3983, 1 ("dimension size")) -> (w3982:T23)
              n576 = Initialize Array(w3996, 1 ("dimension size")) -> (w3992:cluster{sgl, sgl}[])
              n577 = Insert Into Array(array=w3990, index=w3989, new element=w3988) -> (w3987:dbl[])
              n578 = Array Max & Min(array=w3987) -> (max value=w3980:dbl)  [unwired: 3 out]
              n579 = Divide(x=w3980, y=0.9) -> (x/y=w3971:dbl)
              n580 = property on="maximum" class="DigNum (strict)"("Val(Sgnl)"=w3971) -> ()  [unwired: 2 in, 2 out]
              n581 = call <vilib>:"Polar Plot(points&line).vi"("polar attributes"="polar attributes", "desired font(Application)"=w4002, "dimensions (w,h)"=w4004, "data array [mag, phase (deg)]"=w4003) -> ("new picture"=w3999:picture)  [unwired: 7 in]
              n582 = property on="maximum" class="DigNum (strict)"("Val(Sgnl)"=w3971) -> ()  [unwired: 2 in, 2 out]
              n583 = property on="maximum" class="DigNum (strict)"("Val(Sgnl)"=w3971) -> ()  [unwired: 2 in, 2 out]
              n584 = property on="maximum" class="DigNum (strict)"("Val(Sgnl)"=w3971) -> ()  [unwired: 2 in, 2 out]
              n585 = feedback #1() -> (w3998:picture)  [unwired: 1 in]
              n586 = call <vilib>:"Polar Plot(points&line).vi"("polar attributes"="polar attributes Prediction", "desired font(Application)"=w4002, "dimensions (w,h)"=w4004, "data array [mag, phase (deg)]"=w3982, "picture"=w3998) -> ("new picture"=w3986:picture)  [unwired: 6 in]
              n587 = call <vilib>:"Polar Plot(points&line).vi"("polar attributes"="polar attributes Start Point", "desired font(Application)"=w4002, "dimensions (w,h)"=w4004, "data array [mag, phase (deg)]"=w3992, "picture"=w3986) -> ("new picture"=w3973:picture)  [unwired: 6 in]
              n588 = call <vilib>:"Polar Plot(points&line).vi"("polar attributes"="polar attributes Marker", "desired font(Application)"=w4002, "dimensions (w,h)"=w4004, "data array [mag, phase (deg)]"=w3967, "picture"=w3973) -> ("new picture"=→"Polar Plot Picture":picture)  [unwired: 6 in]
              n589 = feedback-in #1(w3999) -> ()
            }
          }
          n590 = local read "Ship Class"() -> (w3555:T4)
          n591 = local read "Frequency (Hz) 1"() -> (w3556:dbl)
          n592 = case shown="\"LA Class\"" w3555 {
            tunnel: w3407 -> [w4856 w4871 w4872]
            tunnel: [w4842 w4857 w4874] -> w3457
            tunnel: [w4855 w4870 w4873] -> w3477
            frame "LA Class" {
              n593 = Split Signals(w4856) -> (w4855:dynamicdata, w4854:dynamicdata, w4853:dynamicdata, w4852:dynamicdata, w4851:dynamicdata, w4850:dynamicdata, w4849:dynamicdata, w4848:dynamicdata, w4847:dynamicdata, w4846:dynamicdata, w4845:dynamicdata, w4844:dynamicdata, w4843:dynamicdata)  [unwired: 13 in]
              n594 = Merge Signals(w4854, w4853, w4852, w4851, w4850, w4849, w4848, w4847, w4846, w4845, w4844, w4843) -> (w4842:dynamicdata)
            }
            frame "Ohio Class" {
              n595 = Split Signals(w4871) -> (w4870:dynamicdata, w4869:dynamicdata, w4868:dynamicdata, w4867:dynamicdata, w4866:dynamicdata, w4865:dynamicdata, w4864:dynamicdata, w4863:dynamicdata, w4862:dynamicdata, w4861:dynamicdata, w4860:dynamicdata, w4859:dynamicdata, w4858:dynamicdata)  [unwired: 13 in]
              n596 = Merge Signals(w4869, w4868, w4867, w4866, w4865, w4864, w4863, w4862, w4861, w4860, w4859, w4858) -> (w4857:dynamicdata)
            }
            frame "Simulated Signals Ohio" {
              n597 = Split Signals(w4872) -> (w4873:dynamicdata, w4875:dynamicdata, w4876:dynamicdata, w4877:dynamicdata, w4878:dynamicdata, w4879:dynamicdata, w4880:dynamicdata, w4881:dynamicdata, w4882:dynamicdata, w4883:dynamicdata)  [unwired: 10 in]
              n598 = Merge Signals(w4875, w4876, w4877, w4878, w4879, w4880, w4881, w4882, w4883) -> (w4874:dynamicdata)
            }
          }
          n599 = local read "Sample Frequency (Hz)"() -> (w3528:i32)
          n600 = local read "Sample Frequency (Hz)"() -> (w3529:i32)
          n601 = local read "Sample Frequency (Hz)"() -> (w3527:i32)
          n602 = local read "Sample Frequency (Hz)"() -> (w3482:i32)
          n603 = case shown="\"Simulated Signals Ohio\"" w3555 {
            tunnel: w3406 -> [w4803 w4826 w4841]
            tunnel: [w4802 w4812 w4827] -> w3665
            tunnel: [w4801 w4825 w4840] -> w3666
            frame "Simulated Signals Ohio" {
              n604 = Split Signals(w4803) -> (w4801:dynamicdata, w4804:dynamicdata, w4805:dynamicdata, w4806:dynamicdata, w4807:dynamicdata, w4808:dynamicdata, w4809:dynamicdata, w4810:dynamicdata, w4811:dynamicdata, w4800:dynamicdata)  [unwired: 10 in]
              n605 = Merge Signals(w4804, w4805, w4806, w4807, w4808, w4809, w4810, w4811, w4800) -> (w4802:dynamicdata)
            }
            frame "LA Class" {
              n606 = Split Signals(w4826) -> (w4825:dynamicdata, w4824:dynamicdata, w4823:dynamicdata, w4822:dynamicdata, w4821:dynamicdata, w4820:dynamicdata, w4819:dynamicdata, w4818:dynamicdata, w4817:dynamicdata, w4816:dynamicdata, w4815:dynamicdata, w4814:dynamicdata, w4813:dynamicdata)  [unwired: 13 in]
              n607 = Merge Signals(w4824, w4823, w4822, w4821, w4820, w4819, w4818, w4817, w4816, w4815, w4814, w4813) -> (w4812:dynamicdata)
            }
            frame "Ohio Class" {
              n608 = Split Signals(w4841) -> (w4840:dynamicdata, w4839:dynamicdata, w4838:dynamicdata, w4837:dynamicdata, w4836:dynamicdata, w4835:dynamicdata, w4834:dynamicdata, w4833:dynamicdata, w4832:dynamicdata, w4831:dynamicdata, w4830:dynamicdata, w4829:dynamicdata, w4828:dynamicdata)  [unwired: 13 in]
              n609 = Merge Signals(w4839, w4838, w4837, w4836, w4835, w4834, w4833, w4832, w4831, w4830, w4829, w4828) -> (w4827:dynamicdata)
            }
          }
          n610 = local read "Frequency (Hz) 2"() -> (w3557:dbl)
          n611 = local read "Frequency (Hz) 1"() -> (w3643:dbl)
          n612 = local read "Frequency (Hz) 2"() -> (w3483:dbl)
          n613 = Array Size(array=w3523) -> (size(s)=w3520:i32)
          n614 = Array Size(array=w3478) -> (size(s)=w3531:i32)
          n615 = Decrement(x=w3520) -> (x-1=w3519:i32)
          n616 = Decrement(x=w3531) -> (x-1=w3521:i32)
          n617 = Array Size(array=w3480) -> (size(s)=w3571:i32)
          n618 = Array Size(array=w3480) -> (size(s)=w3481:i32)
          n619 = for "Phase (Degrees)" {
            N: w3519 -> [_]
            tunnel: w3406 -> [w4979]
            tunnel: [w4981] -> w3691 mode=indexing
            tunnel: w3528 -> [w4980]
            i -> [w4984]
            n620 = Add(x=1, y=w4984) -> (x+y=w4982:i32)
            n621 = call "Convert from Dynamic Data30"("Dynamic Data Type"=w4979, "Channel"=w4982) -> ("Array"=w4987:dbl[])  [unwired: 2 in]
            n622 = call "Convert from Dynamic Data31"("Dynamic Data Type"=w4979, "Channel"=0) -> ("Array"=w4985:dbl[])  [unwired: 2 in]
            n623 = Reciprocal(x=w4980) -> (1/x=w4991:dbl)
            n624 = call <vilib>:"Cross Power Spectrum.vi"("dt"=w4991, "Signal Y (V)"=w4987, "Signal X (V)"=w4985) -> ("Cross Power XY Spectrum Phase (radians)"=w4978:dbl[])  [unwired: 2 out]
            n625 = Divide(x=180, y=3.141592653589793) -> (x/y=w4988:dbl)
            n626 = Multiply(x=w4978, y=w4988) -> (x*y=w4981:dbl[])
          }
          n627 = for "Magnitude (VdB)" {
            N: w3521 -> [_]
            tunnel: w3478 -> [w5053]
            tunnel: [w5049] -> w3704 mode=indexing
            i -> [w5052]
            n628 = Add(x=1, y=w5052) -> (x+y=w5050:i32)
            n629 = Index Array(array=w5053, index=w5050) -> (element=w5054:cluster{"x0":dbl, "dx":dbl, "magnitude":dbl[]})
            n630 = Unbundle(w5054) -> ("magnitude"=w5049:dbl[])  [unwired: 2 out]
          }
          n631 = Index Array(array=w3478) -> (element=w3705:cluster{"x0":dbl, "dx":dbl, "magnitude":dbl[]})  [unwired: 1 in]
          n632 = for "Phase (Degrees)" {
            N: w3521 -> [_]
            tunnel: w3407 -> [w5091]
            tunnel: [w5087] -> w3559 mode=indexing
            tunnel: w3529 -> [w5085]
            i -> [w5089]
            n633 = Add(x=1, y=w5089) -> (x+y=w5086:i32)
            n634 = call "Convert from Dynamic Data27"("Dynamic Data Type"=w5091, "Channel"=w5086) -> ("Array"=w5093:dbl[])  [unwired: 2 in]
            n635 = call "Convert from Dynamic Data28"("Dynamic Data Type"=w5091, "Channel"=0) -> ("Array"=w5090:dbl[])  [unwired: 2 in]
            n636 = Reciprocal(x=w5085) -> (1/x=w5098:dbl)
            n637 = call <vilib>:"Cross Power Spectrum.vi"("dt"=w5098, "Signal Y (V)"=w5093, "Signal X (V)"=w5090) -> ("Cross Power XY Spectrum Phase (radians)"=w5097:dbl[])  [unwired: 2 out]
            n638 = Divide(x=180, y=3.141592653589793) -> (x/y=w5094:dbl)
            n639 = Multiply(x=w5097, y=w5094) -> (x*y=w5087:dbl[])
          }
          n640 = for "Magnitude (VdB)" {
            N: w3519 -> [_]
            tunnel: w3523 -> [w4945]
            tunnel: [w4941] -> w3689 mode=indexing
            i -> [w4944]
            n641 = Add(x=1, y=w4944) -> (x+y=w4942:i32)
            n642 = Index Array(array=w4945, index=w4942) -> (element=w4946:cluster{"x0":dbl, "dx":dbl, "magnitude":dbl[]})
            n643 = Unbundle(w4946) -> ("magnitude"=w4941:dbl[])  [unwired: 2 out]
          }
          n644 = Index Array(array=w3523) -> (element=w3690:cluster{"x0":dbl, "dx":dbl, "magnitude":dbl[]})  [unwired: 1 in]
          n645 = for "Magnitude (VdB)" {
            N: w3571 -> [_]
            tunnel: w3480 -> [w4754]
            tunnel: [w4753] -> w3662 mode=indexing
            i -> [w4752]
            n646 = Index Array(array=w4754, index=w4752) -> (element=w4755:cluster{"x0":dbl, "dx":dbl, "magnitude":dbl[]})
            n647 = Unbundle(w4755) -> ("magnitude"=w4753:dbl[])  [unwired: 2 out]
          }
          n648 = Unbundle(w3705) -> ("dx"=w3703:dbl)  [unwired: 2 out]
          "frequency resolution" <- w3703
          n649 = Index Array(array=w3480) -> (element=w3663:cluster{"x0":dbl, "dx":dbl, "magnitude":dbl[]})  [unwired: 1 in]
          n650 = for "Phase (Degrees)" {
            N: w3571 -> [_]
            tunnel: w3456 -> [w4792]
            tunnel: [w4790] -> w3664 mode=indexing
            tunnel: w3407 -> [w4788]
            tunnel: w3527 -> [w4787]
            i -> [w4789]
            n651 = call "Convert from Dynamic Data33"("Dynamic Data Type"=w4792, "Channel"=w4789) -> ("Array"=w4794:dbl[])  [unwired: 2 in]
            n652 = call "Convert from Dynamic Data34"("Dynamic Data Type"=w4788, "Channel"=0) -> ("Array"=w4791:dbl[])  [unwired: 2 in]
            n653 = Reciprocal(x=w4787) -> (1/x=w4799:dbl)
            n654 = call <vilib>:"Cross Power Spectrum.vi"("dt"=w4799, "Signal Y (V)"=w4794, "Signal X (V)"=w4791) -> ("Cross Power XY Spectrum Phase (radians)"=w4798:dbl[])  [unwired: 2 out]
            n655 = Divide(x=180, y=3.141592653589793) -> (x/y=w4795:dbl)
            n656 = Multiply(x=w4798, y=w4795) -> (x*y=w4790:dbl[])
          }
          n657 = Unbundle(w3690) -> ("dx"=w3688:dbl)  [unwired: 2 out]
          n658 = for "Magnitude (VdB)" {
            N: w3481 -> [_]
            tunnel: w3480 -> [w4307]
            tunnel: [w4306] -> w3513 mode=indexing
            i -> [w4305]
            n659 = Index Array(array=w4307, index=w4305) -> (element=w4308:cluster{"x0":dbl, "dx":dbl, "magnitude":dbl[]})
            n660 = Unbundle(w4308) -> ("magnitude"=w4306:dbl[])  [unwired: 2 out]
          }
          n661 = Index Array(array=w3480) -> (element=w3514:cluster{"x0":dbl, "dx":dbl, "magnitude":dbl[]})  [unwired: 1 in]
          n662 = for "Phase (Degrees)" {
            N: w3481 -> [_]
            tunnel: w3456 -> [w4345]
            tunnel: [w4343] -> w3515 mode=indexing
            tunnel: w3406 -> [w4341]
            tunnel: w3482 -> [w4340]
            i -> [w4342]
            n663 = call "Convert from Dynamic Data"("Dynamic Data Type"=w4345, "Channel"=w4342) -> ("Array"=w4347:dbl[])  [unwired: 2 in]
            n664 = call "Convert from Dynamic Data2"("Dynamic Data Type"=w4341, "Channel"=0) -> ("Array"=w4344:dbl[])  [unwired: 2 in]
            n665 = Reciprocal(x=w4340) -> (1/x=w4352:dbl)
            n666 = call <vilib>:"Cross Power Spectrum.vi"("dt"=w4352, "Signal Y (V)"=w4347, "Signal X (V)"=w4344) -> ("Cross Power XY Spectrum Phase (radians)"=w4351:dbl[])  [unwired: 2 out]
            n667 = Divide(x=180, y=3.141592653589793) -> (x/y=w4348:dbl)
            n668 = Multiply(x=w4351, y=w4348) -> (x*y=w4343:dbl[])
          }
          n669 = Unbundle(w3663) -> ("dx"=w3661:dbl)  [unwired: 2 out]
          "frequency (resolution) corner" <- w3661
          n670 = Unbundle(w3514) -> ("dx"=w3512:dbl)  [unwired: 2 out]
          "frequency (resolution) corners-port" <- w3512
          n671 = for "Mag (VdB)(8x)" {
            N: w3521 -> [_]
            tunnel: w3704 -> [w5035]
            tunnel: w3703 -> [w5033]
            tunnel: w3556 -> [w5031]
            tunnel: [w5030] -> w3696 mode=indexing
            i -> [w5032]
            n672 = Index Array(array=w5035, index (row)=w5032) -> (element=w5029:dbl[])  [unwired: 1 in]
            n673 = for {
              N: 8 -> [_]
              tunnel: [w5040] -> w5030 mode=indexing
              tunnel: w5029 -> [w5044]
              tunnel: w5031 -> [w5046]
              tunnel: w5033 -> [w5048]
              i -> [w5045]
              w5038 = ext 2.0  # change
              n674 = Divide(x=w5046, y=w5048) -> (x/y=w5036:dbl)
              n675 = Multiply(x=w5036, y=w5045) -> (x*y=w5047:dbl)
              n676 = Add(x=w5036, y=w5047) -> (x+y=w5042:dbl)
              n677 = Subtract(x=w5042, y=w5038) -> (x-y=w5043:ext)
              n678 = Multiply(x=w5038, y=2.0) -> (x*y=w5037:ext)
              n679 = Array Subset(array=w5044, index=w5043, length=w5037) -> (w5041:dbl[])
              n680 = Array Max & Min(array=w5041) -> (max value=w5040:dbl)  [unwired: 3 out]
            }
          }
          "Magnitude VdB Stbd" <- w3696
          n681 = for "Mag (VdB)(8x)" {
            N: w3519 -> [_]
            tunnel: w3689 -> [w4927]
            tunnel: w3688 -> [w4925]
            tunnel: w3557 -> [w4923]
            tunnel: [w4922] -> w3681 mode=indexing
            i -> [w4924]
            n682 = Index Array(array=w4927, index (row)=w4924) -> (element=w4921:dbl[])  [unwired: 1 in]
            n683 = for {
              N: 8 -> [_]
              tunnel: [w4932] -> w4922 mode=indexing
              tunnel: w4921 -> [w4936]
              tunnel: w4923 -> [w4938]
              tunnel: w4925 -> [w4940]
              i -> [w4937]
              w4930 = ext 2.0  # change
              n684 = Divide(x=w4938, y=w4940) -> (x/y=w4928:dbl)
              n685 = Multiply(x=w4928, y=w4937) -> (x*y=w4939:dbl)
              n686 = Add(x=w4928, y=w4939) -> (x+y=w4934:dbl)
              n687 = Subtract(x=w4934, y=w4930) -> (x-y=w4935:ext)
              n688 = Multiply(x=w4930, y=2.0) -> (x*y=w4929:ext)
              n689 = Array Subset(array=w4936, index=w4935, length=w4929) -> (w4933:dbl[])
              n690 = Array Max & Min(array=w4933) -> (max value=w4932:dbl)  [unwired: 3 out]
            }
          }
          "Magnitude VdB Port" <- w3681
          n691 = for "Mag (VdB)(8x)" {
            N: w3571 -> [_]
            tunnel: w3662 -> [w4739]
            tunnel: w3661 -> [w4737]
            tunnel: w3643 -> [w4735]
            tunnel: [w4734] -> w3644 mode=indexing
            i -> [w4736]
            n692 = Index Array(array=w4739, index (row)=w4736) -> (element=w4733:dbl[])  [unwired: 1 in]
            n693 = for {
              N: 8 -> [_]
              tunnel: [w4745] -> w4734 mode=indexing
              tunnel: w4733 -> [w4747]
              tunnel: w4735 -> [w4749]
              tunnel: w4737 -> [w4751]
              i -> [w4748]
              # "Encompass wider span\nto ensure max capture"
              n694 = Divide(x=w4749, y=w4751) -> (x/y=w4743:dbl)
              n695 = Multiply(x=w4743, y=w4748) -> (x*y=w4750:dbl)
              n696 = Add(x=w4743, y=w4750) -> (x+y=w4742:dbl)
              n697 = Subtract(x=w4742, y=1 ("length")) -> (x-y=w4740:dbl)
              n698 = Array Subset(array=w4747, index=w4740, length=3) -> (w4746:dbl[])
              n699 = Array Max & Min(array=w4746) -> (max value=w4745:dbl)  [unwired: 3 out]
            }
          }
          "Magnitude VdB Corner" <- w3644
          n700 = for "Mag (VdB)(8x)" {
            N: w3481 -> [_]
            tunnel: w3513 -> [w4290]
            tunnel: w3512 -> [w4288]
            tunnel: w3483 -> [w4286]
            tunnel: [w4285] -> w3495 mode=indexing
            i -> [w4287]
            n701 = Index Array(array=w4290, index (row)=w4287) -> (element=w4284:dbl[])  [unwired: 1 in]
            n702 = for {
              N: 8 -> [_]
              tunnel: [w4298] -> w4285 mode=indexing
              tunnel: w4284 -> [w4300]
              tunnel: w4286 -> [w4302]
              tunnel: w4288 -> [w4304]
              i -> [w4301]
              n703 = Divide(x=w4302, y=w4304) -> (x/y=w4297:dbl)
              n704 = Multiply(x=w4297, y=w4301) -> (x*y=w4303:dbl)
              n705 = Subtract(x=w4297, y=1.0) -> (x-y=w4295:dbl)
              n706 = Add(x=w4295, y=w4303) -> (x+y=w4292:dbl)
              n707 = Subtract(x=w4292, y=1 ("length")) -> (x-y=w4291:dbl)
              n708 = Array Subset(array=w4300, index=w4291, length=3) -> (w4299:dbl[])
              n709 = Array Max & Min(array=w4299) -> (max value=w4298:dbl)  [unwired: 3 out]
            }
          }
          "Magnitude VdB Corners-Port" <- w3495
          n710 = for "Phase (8x)" {
            N: w3521 -> [_]
            tunnel: w3559 -> [w5061]
            tunnel: [w5057] -> w3558 mode=indexing
            tunnel: w3556 -> [w5056]
            tunnel: w3703 -> [w5055]
            i -> [w5058]
            n711 = Index Array(array=w5061, index (row)=w5058) -> (element=w5059:dbl[])  [unwired: 1 in]
            n712 = for {
              N: 8 -> [_]
              tunnel: [w5067] -> w5057 mode=indexing
              tunnel: w5059 -> [w5069]
              tunnel: w5056 -> [w5065]
              tunnel: w5055 -> [w5064]
              i -> [w5070]
              n713 = Divide(x=w5065, y=w5064) -> (x/y=w5063:dbl)
              n714 = Multiply(x=w5063, y=w5070) -> (x*y=w5071:dbl)
              n715 = Add(x=w5063, y=w5071) -> (x+y=w5068:dbl)
              n716 = Index Array(array=w5069, index=w5068) -> (element=w5062:dbl)
              n717 = case shown="\"navbal\"" "phase data format" {
                tunnel: w5062 -> [w5076 w5079 w5084]
                tunnel: [w5072 w5078 w5084] -> w5067
                frame "0-360" {
                  n718 = Negate(x=w5076) -> (-x=w5074:dbl)
                  n719 = Less Than 0?(x=w5076) -> (x < 0?=w5077:bool)
                  n720 = Add(x=w5074, y=180.0) -> (x+y=w5073:dbl)
                  n721 = Select(t=w5073, s=w5077, f=w5076) -> (s? t:f=w5072:dbl)
                }
                frame "navbal" {
                  n722 = Negate(x=w5079) -> (-x=w5083:dbl)
                  n723 = Less Than 0?(x=w5079) -> (x < 0?=w5082:bool)
                  n724 = Subtract(x=360.0, y=w5079) -> (x-y=w5081:dbl)
                  n725 = Select(t=w5083, s=w5082, f=w5081) -> (s? t:f=w5078:dbl)
                }
                frame "pass through", Default {
                }
              }
            }
          }
          "Phase Stbd" <- w3558
          n726 = local read "phase data format"() -> (w3517:string)
          n727 = for "Phase (8x)" {
            N: w3519 -> [_]
            tunnel: w3691 -> [w4954]
            tunnel: [w4950] -> w3415 mode=indexing
            tunnel: w3557 -> [w4949]
            tunnel: w3688 -> [w4948]
            tunnel: w3517 -> [w4947]
            i -> [w4951]
            n728 = Index Array(array=w4954, index (row)=w4951) -> (element=w4952:dbl[])  [unwired: 1 in]
            n729 = for {
              N: 8 -> [_]
              tunnel: [w4959] -> w4950 mode=indexing
              tunnel: w4952 -> [w4962]
              tunnel: w4949 -> [w4958]
              tunnel: w4948 -> [w4957]
              tunnel: w4947 -> [w4955]
              i -> [w4963]
              n730 = Divide(x=w4958, y=w4957) -> (x/y=w4956:dbl)
              n731 = Multiply(x=w4956, y=w4963) -> (x*y=w4964:dbl)
              n732 = Add(x=w4956, y=w4964) -> (x+y=w4961:dbl)
              n733 = Index Array(array=w4962, index=w4961) -> (element=w4960:dbl)
              n734 = case shown="\"navbal\"" w4955 {
                tunnel: w4960 -> [w4969 w4972 w4977]
                tunnel: [w4965 w4971 w4977] -> w4959
                frame "0-360" {
                  n735 = Negate(x=w4969) -> (-x=w4967:dbl)
                  n736 = Less Than 0?(x=w4969) -> (x < 0?=w4970:bool)
                  n737 = Add(x=w4967, y=180.0) -> (x+y=w4966:dbl)
                  n738 = Select(t=w4966, s=w4970, f=w4969) -> (s? t:f=w4965:dbl)
                }
                frame "navbal" {
                  n739 = Negate(x=w4972) -> (-x=w4976:dbl)
                  n740 = Less Than 0?(x=w4972) -> (x < 0?=w4975:bool)
                  n741 = Subtract(x=360.0, y=w4972) -> (x-y=w4974:dbl)
                  n742 = Select(t=w4976, s=w4975, f=w4974) -> (s? t:f=w4971:dbl)
                }
                frame "pass through", Default {
                }
              }
            }
          }
          "Phase Port" <- w3415
          n743 = local read "Port/Starboard"() -> (w3329:enum32{"Port Side", "Stbd Side"})
          n744 = local read "phase data format"() -> (w3479:string)
          n745 = for "Phase (8x)" {
            N: w3481 -> [_]
            tunnel: w3515 -> [w4316]
            tunnel: [w4312] -> w3486 mode=indexing
            tunnel: w3483 -> [w4311]
            tunnel: w3512 -> [w4310]
            tunnel: w3479 -> [w4309]
            i -> [w4313]
            n746 = Index Array(array=w4316, index (row)=w4313) -> (element=w4314:dbl[])  [unwired: 1 in]
            n747 = for {
              N: 8 -> [_]
              tunnel: [w4321] -> w4312 mode=indexing
              tunnel: w4314 -> [w4324]
              tunnel: w4311 -> [w4320]
              tunnel: w4310 -> [w4319]
              tunnel: w4309 -> [w4318]
              i -> [w4325]
              n748 = Divide(x=w4320, y=w4319) -> (x/y=w4317:dbl)
              n749 = Multiply(x=w4317, y=w4325) -> (x*y=w4326:dbl)
              n750 = Add(x=w4317, y=w4326) -> (x+y=w4323:dbl)
              n751 = Index Array(array=w4324, index=w4323) -> (element=w4322:dbl)
              n752 = case shown="\"navbal\"" w4318 {
                tunnel: w4322 -> [w4331 w4334 w4339]
                tunnel: [w4327 w4333 w4339] -> w4321
                frame "0-360" {
                  n753 = Negate(x=w4331) -> (-x=w4329:dbl)
                  n754 = Less Than 0?(x=w4331) -> (x < 0?=w4332:bool)
                  n755 = Add(x=w4329, y=180.0) -> (x+y=w4328:dbl)
                  n756 = Select(t=w4328, s=w4332, f=w4331) -> (s? t:f=w4327:dbl)
                }
                frame "navbal" {
                  n757 = Negate(x=w4334) -> (-x=w4338:dbl)
                  n758 = Less Than 0?(x=w4334) -> (x < 0?=w4337:bool)
                  n759 = Subtract(x=360.0, y=w4334) -> (x-y=w4336:dbl)
                  n760 = Select(t=w4338, s=w4337, f=w4336) -> (s? t:f=w4333:dbl)
                }
                frame "pass through", Default {
                }
              }
            }
          }
          "Phase Corner 2" <- w3486
          n761 = property on="Boat File" class="Path"() -> ("Value"=w3337:path)  [unwired: 2 in, 2 out]
          n762 = local read "phase data format"() -> (w3516:string)
          n763 = for "Phase (8x)" {
            N: w3571 -> [_]
            tunnel: w3664 -> [w4763]
            tunnel: [w4759] -> w3618 mode=indexing
            tunnel: w3643 -> [w4758]
            tunnel: w3661 -> [w4757]
            tunnel: w3516 -> [w4756]
            i -> [w4760]
            n764 = Index Array(array=w4763, index (row)=w4760) -> (element=w4761:dbl[])  [unwired: 1 in]
            n765 = for {
              N: 8 -> [_]
              tunnel: [w4768] -> w4759 mode=indexing
              tunnel: w4761 -> [w4771]
              tunnel: w4758 -> [w4767]
              tunnel: w4757 -> [w4766]
              tunnel: w4756 -> [w4765]
              i -> [w4772]
              n766 = Divide(x=w4767, y=w4766) -> (x/y=w4764:dbl)
              n767 = Multiply(x=w4764, y=w4772) -> (x*y=w4773:dbl)
              n768 = Add(x=w4764, y=w4773) -> (x+y=w4770:dbl)
              n769 = Index Array(array=w4771, index=w4770) -> (element=w4769:dbl)
              n770 = case shown="\"navbal\"" w4765 {
                tunnel: w4769 -> [w4778 w4781 w4786]
                tunnel: [w4774 w4780 w4786] -> w4768
                frame "0-360" {
                  n771 = Negate(x=w4778) -> (-x=w4776:dbl)
                  n772 = Less Than 0?(x=w4778) -> (x < 0?=w4779:bool)
                  n773 = Add(x=w4776, y=180.0) -> (x+y=w4775:dbl)
                  n774 = Select(t=w4775, s=w4779, f=w4778) -> (s? t:f=w4774:dbl)
                }
                frame "navbal" {
                  n775 = Negate(x=w4781) -> (-x=w4785:dbl)
                  n776 = Less Than 0?(x=w4781) -> (x < 0?=w4784:bool)
                  n777 = Subtract(x=360.0, y=w4781) -> (x-y=w4783:dbl)
                  n778 = Select(t=w4785, s=w4784, f=w4783) -> (s? t:f=w4780:dbl)
                }
                frame "pass through", Default {
                }
              }
            }
          }
          "Phase Corner" <- w3618
          n779 = case "Pick out Mag, Phase, and Weight locations from Excel File" shown="True" "Slct Strt Pt" {
            tunnel: "Marker Listbox" -> [_ w3714]
            tunnel: w3337 -> [_ w3728]
            tunnel: w3329 -> [_ w3711]
            frame False {
            }
            frame True {
              n780 = property on="Marker Listbox" class="MCListbox (strict)"() -> ("ItemNames"=w3713:string[][])  [unwired: 2 in, 2 out]
              n781 = case shown="\"Stbd Side\"" w3711 {
                tunnel: [w3768 w3770] -> w3719
                tunnel: [4 ("y") 5 ("x")] -> w3708
                frame "Port Side", Default {
                  n782 = local read "#Stbd Accels"() -> (w3768:i32)
                }
                frame "Stbd Side" {
                  n783 = local read "#Port Accels"() -> (w3770:i32)
                }
              }
              n784 = Multiply(x=w3714, y=2) -> (x*y=w3726:i32)
              n785 = Increment(x=w3726) -> (x+1=w3724:i32)
              n786 = Index Array(array=w3713, index (row)=w3714, index (col)=0 ("disabled index (col)")) -> (element=→"Indicate Ref":string)
              n787 = call <vilib>:"New Report.vi"("report type"=T11."Excel", "template (empty)"=w3728) -> ("report out"=w3734:refnum<class "NI_report.lvclass">, "error out"=w3735:errorcluster)  [unwired: 12 in]
              n788 = Bundle("y"=12, w3724) -> (w3731:cluster{"y":i32, i32})  [unwired: 1 in]
              n789 = call <vilib>:"Excel Get Worksheet.vi"("report in"=w3734, "worksheet index (0)"=w3708, "error in (no error)"=w3735) -> ("report out"=w3737:refnum<class "NI_report.lvclass">, "error out"=w3738:errorcluster)  [unwired: 11 out]
              n790 = local read "#Corner Accels"() -> (w3718:i32)
